vi "Add.vi"(8 "Error In":errorcluster, 10 "Component":refnum<class "MenuComponent.lvclass">, 11 "reference in":refnum<class "Menu.lvclass">) -> (0 "Error Out":errorcluster, 3 "reference in":refnum<class "Menu.lvclass">)   [LabVIEW 2020, in "Menu.lvclass"]
uses:
  Menu.lvclass
  MenuComponent_class/MenuComponent.lvclass
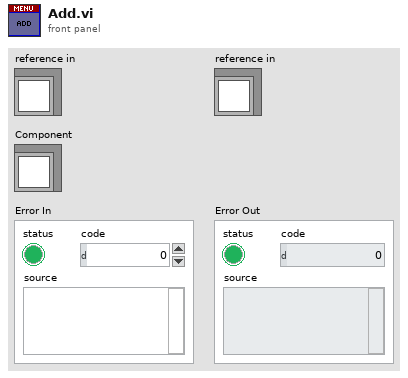
[diagram p1: front panel]
types:
  T1 = typedef "Menu.lvclass/ObjectAttributes.ctl" = cluster{"Items":refnum<class "MenuComponent.lvclass">[], "Name":string, "Description":string}
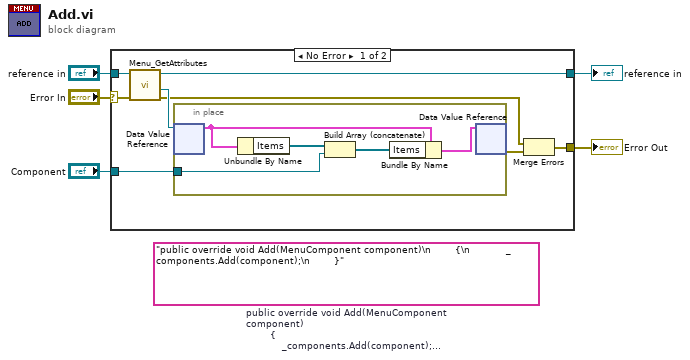
[diagram p0: block diagram]
diagram:
  (unwired) "public override void Add(MenuComponent component)\n        {\n            _components.Add(component);\n        }"  # public override void Add(MenuComponent component)         {             _components.Add(component);         }
  n1 = case shown="No Error" "Error In" {
    selector: "Error In" -> [w12 w20]
    tunnel: [w11 w20] -> w4
    tunnel: [w10 w19] -> w2
    tunnel: "reference in" -> [w13 w19]
    tunnel: "Component" -> [w6 _]
    frame No Error {
      n2 = call "Menu_GetAttributes.vi"("error in (no error)"=w12, "reference in"=w13) -> ("error out"=w8:errorcluster, "DataRef"=w9:refnum<data-value>, "reference out"=w10:refnum<class "Menu.lvclass">)  [unwired: 6 in, 1 out]
      n3 = in-place {
        in-place-border: w6 -> [w15]
        n4 = in-place-dvr #1(w9) -> (w17:T1)  [unwired: 1 out]
        n5 = Unbundle By Name(w17) -> ("Items"=w16:refnum<class "MenuComponent.lvclass">[])
        n6 = Build Array (concatenate)(w16, w15) -> (w14:refnum<class "MenuComponent.lvclass">[])
        n7 = Bundle By Name(cluster=w17, "Items"=w14) -> (w18:T1)
        n8 = in-place-dvr #1(w18) -> (w7:errorcluster)  [unwired: 1 out]
      }
      n9 = Merge Errors(w8, w7) -> (w11:errorcluster)
    }
    frame Error {
    }
  }
  "Error Out" <- w4
  "reference in" <- w2
